vi "insert or remove logger.vi"(5 "action":T1, 6 "timeout (1000) [ms]":u32=1000, 7 "handler name":string, 8 "error in (no error)":errorcluster, 11 "handler to insert":refnum<class "Handler.lvclass">) -> (0 "error out":errorcluster)   [LabVIEW 2024, in "status manager.lvlib"]
uses:
  status manager.lvlib
  <vilib>/Hampel Software Engineering/HSE Logger/Handler/Handler.lvclass
  logger actions.ctl
  <vilib>/Hampel Software Engineering/HSE Logger/Logger/Logger.lvclass
  <vilib>/Hampel Software Engineering/HSE Logger/hse-logger.lvlib
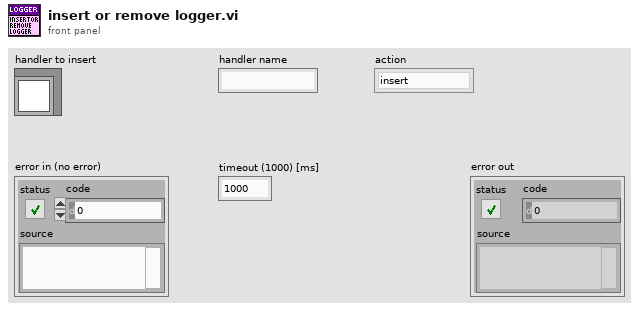
[diagram p1: front panel]
types:
  T1 = typedef "status manager.lvlib/logger actions.ctl" = enum16{"insert", "remove"}
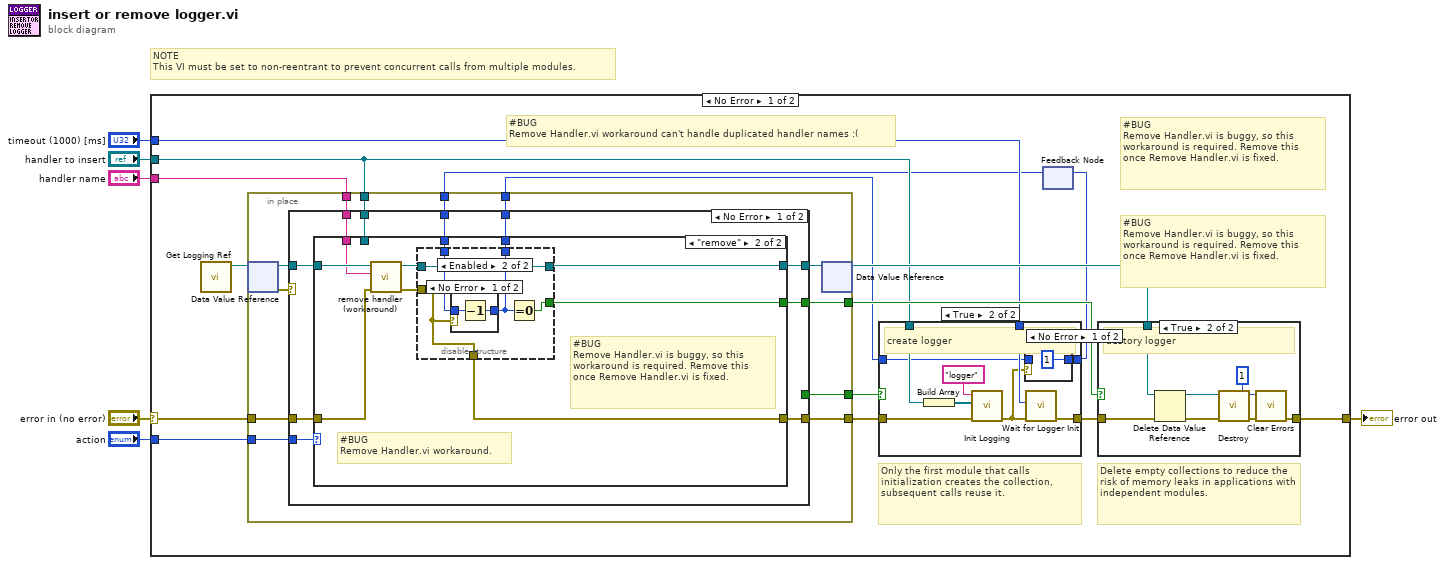
[diagram p0: block diagram]
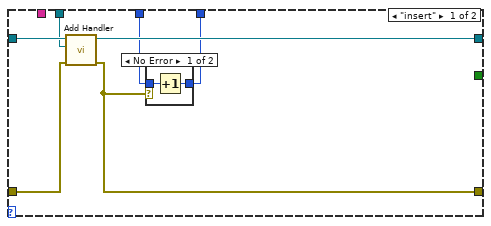
[diagram p3: hidden frame]
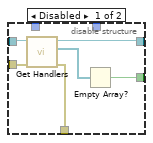
[diagram p5: hidden frame]
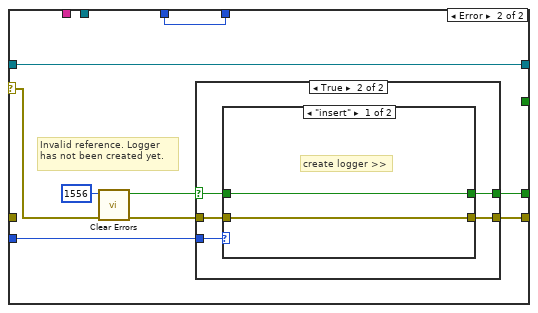
[diagram p7: hidden frame]
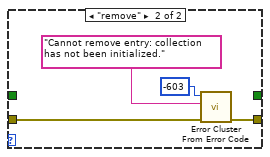
[diagram p9: hidden frame]
diagram:
  # "NOTE\nThis VI must be set to non-reentrant to prevent concurrent calls from multiple modules."
  n1 = case shown="No Error" "error in (no error)" {
    selector: "error in (no error)" -> [w14 w120]
    tunnel: [w11 w120] -> w6
    tunnel: "handler to insert" -> [w17 _]
    tunnel: "timeout (1000) [ms]" -> [w16 _]
    tunnel: "action" -> [w15 _]
    tunnel: "handler name" -> [w13 _]
    frame No Error {
      # "#BUG\nRemove Handler.vi workaround can't handle duplicated handler names :("
      # "#BUG\nRemove Handler.vi is buggy, so this workaround is required. Remove this once Remove Handler.vi is fixed."
      # "#BUG\nRemove Handler.vi is buggy, so this workaround is required. Remove this once Remove Handler.vi is fixed."
      # "Only the first module that calls initialization creates the collection, subsequent calls reuse it."
      # "Delete empty collections to reduce the risk of memory leaks in applications with independent modules."
      n2 = call <vilib>:"Get Logging Ref.vi"() -> ("Logger DVR"=w19:refnum<data-value>)  [unwired: 10 in, 1 out]
      n3 = feedback #1() -> (w7:u32)  [unwired: 1 in]
      n4 = in-place {
        in-place-border: [w38] -> w10
        in-place-border: [w37] -> w18
        in-place-border: w17 -> [w36]
        in-place-border: w15 -> [w35]
        in-place-border: w14 -> [w34]
        in-place-border: w13 -> [w33]
        in-place-border: [w32] -> w20
        in-place-border: [w31] -> w9
        in-place-border: w7 -> [w30]
        n5 = in-place-dvr #2(w19) -> (w40:refnum<class "Logger.lvclass">, w41:errorcluster)
        n6 = case shown="No Error" w41 {
          selector: w41 -> [_ w93]
          tunnel: w40 -> [w51 w94]
          tunnel: [w50 w94] -> w39
          tunnel: [w48 w90] -> w38
          tunnel: [_ w87] -> w37
          tunnel: w36 -> [w49 _]
          tunnel: w35 -> [w47 w89]
          tunnel: w34 -> [w46 _]
          tunnel: w33 -> [w45 _]
          tunnel: [w44 _] -> w32
          tunnel: [w43 w86] -> w31
          tunnel: w30 -> [w42 w86]
          frame No Error {
            n7 = case shown="\"remove\"" w47 {
              tunnel: w51 -> [w58 w70]
              tunnel: [w57 w69] -> w50
              tunnel: w49 -> [w56 _]
              tunnel: [w52 w66] -> w48
              tunnel: w46 -> [w55 w67]
              tunnel: w45 -> [_ w65]
              tunnel: [_ w64] -> w44
              tunnel: [w53 w63] -> w43
              tunnel: w42 -> [w54 w62]
              frame "insert" {
                n8 = call <vilib>:"Add Handler.vi"("error in"=w55, "Handler"=w56, "Logger in"=w58) -> ("error out"=w52:errorcluster, "Logger out"=w57:refnum<class "Logger.lvclass">)  [unwired: 7 in]
                n9 = case shown="No Error" w52 {
                  tunnel: [w60 w61] -> w53
                  tunnel: w54 -> [w59 w61]
                  frame No Error {
                    n10 = Increment(x=w59) -> (x+1=w60:u32)
                  }
                  frame Error {
                  }
                }
              }
              frame "remove" {
                # "#BUG\nRemove Handler.vi workaround."
                # "#BUG\nRemove Handler.vi is buggy, so this workaround is required. Remove this once Remove Handler.vi is fixed."
                n11 = call "remove handler (workaround).vi"("error in"=w67, "Name"=w65, "Logger in"=w70) -> ("error out"=w68:errorcluster, "Logger out"=w71:refnum<class "Logger.lvclass">)  [unwired: 7 in]
                n12 = disable-structure shown="Enabled" {
                  disable-tunnel: w71 -> [w77 w82]
                  disable-tunnel: [w76 w82] -> w69
                  disable-tunnel: w68 -> [w75 w81]
                  disable-tunnel: [w74 w81] -> w66
                  disable-tunnel: [w72 w78] -> w64
                  disable-tunnel: [_ w79] -> w63
                  disable-tunnel: w62 -> [_ w80]
                  frame Disabled {
                    n13 = call-dynamic "Get Handlers.vi"("error in"=w75, "Logger in"=w77) -> ("error out"=w74:errorcluster, "Handlers"=w73:refnum<class "Handler.lvclass">[], "Logger out"=w76:refnum<class "Logger.lvclass">)  [unwired: 7 in]
                    n14 = Empty Array?(array=w73) -> (empty?=w72:bool)
                  }
                  frame Enabled {
                    n15 = case shown="No Error" w81 {
                      tunnel: [w84 w85] -> w79
                      tunnel: w80 -> [w83 w85]
                      frame No Error {
                        n16 = Decrement(x=w83) -> (x-1=w84:u32)
                      }
                      frame Error {
                      }
                    }
                    n17 = Equal To 0?(x=w79) -> (x = 0?=w78:bool)
                  }
                }
              }
            }
          }
          frame Error {
            # "Invalid reference. Logger has not been created yet."
            n18 = call <vilib>:"Clear Errors.vi"("error in (no error)"=w93, "specific error code to clear (0: all)"=1556) -> ("error out"=w91:errorcluster, "specific error cleared?"=w88:bool)  [unwired: 4 in]
            n19 = case shown="True" w88 {
              selector: w88 -> [_ w96]
              tunnel: w91 -> [w95 w100]
              tunnel: [w95 w99] -> w90
              tunnel: w89 -> [_ w98]
              tunnel: [_ w97] -> w87
              frame False {
              }
              frame True {
                n20 = case shown="\"insert\"" w98 {
                  tunnel: w100 -> [w102 w106]
                  tunnel: [w102 w105] -> w99
                  tunnel: [w101 _] -> w97
                  tunnel: w96 -> [w101 _]
                  frame "insert" {
                    # "create logger >>"
                  }
                  frame "remove" {
                    n21 = call <vilib>:"Error Cluster From Error Code.vi"("error in (no error)"=w106, "error message (\"\")"="Cannot remove entry: collection has not been initialized.", "error code (0)"=-603) -> ("error out"=w105:errorcluster)  [unwired: 6 in]
                  }
                }
              }
            }
          }
        }
        n22 = in-place-dvr #2(w39) -> (w21:refnum<data-value>)  [unwired: 1 out]
      }
      n23 = case shown="True" w18 {
        tunnel: w10 -> [w108 w116]
        tunnel: [w108 w114] -> w12
        tunnel: w17 -> [_ w115]
        tunnel: w16 -> [_ w113]
        tunnel: w9 -> [w107 w111]
        tunnel: [w107 w109] -> w8
        frame False {
        }
        frame True {
          # "create logger"
          n24 = Build Array(w115) -> (w117:refnum<class "Handler.lvclass">[])
          n25 = call <vilib>:"Init Logging.vi"("error in"=w116, "Handlers"=w117, "Name"="logger") -> ("error out"=w110:errorcluster)  [unwired: 8 in]
          n26 = case shown="No Error" w110 {
            tunnel: [u32 1 w119] -> w109
            tunnel: w111 -> [_ w119]
            frame No Error {
            }
            frame Error {
            }
          }
          n27 = call <vilib>:"Wait for Logger Init.vi"("error in (no error)"=w110, "Timeout (ms)"=w113) -> ("error out"=w114:errorcluster)  [unwired: 9 in]
        }
      }
      n28 = feedback-in #1(w8) -> ()
      n29 = case shown="True" w20 {
        tunnel: w12 -> [w22 w29]
        tunnel: [w22 w24] -> w11
        tunnel: w21 -> [_ w26]
        frame False {
        }
        frame True {
          # "destory logger"
          n30 = Delete Data Value Reference(data value reference=w26, error in=w29) -> (data value=w25:refnum<class "Logger.lvclass">, error out=w28:errorcluster)
          n31 = call-dynamic "Destroy.vi"("error in"=w28, "Logger in"=w25) -> ("error out"=w27:errorcluster)  [unwired: 8 in, 1 out]
          n32 = call <vilib>:"Clear Errors.vi"("error in (no error)"=w27, "specific error code to clear (0: all)"=1) -> ("error out"=w24:errorcluster)  [unwired: 4 in, 1 out]
        }
      }
    }
    frame Error {
    }
  }
  "error out" <- w6
